vi "Tesla_Test.vi"() -> ()   [LabVIEW 2013]
uses:
  MM3_TESLA/Powerboard 1.0/Control/Command Enum.ctl
  <vilib>/Utility/NIReport.llb/NI_report.lvclass
  <vilib>/Utility/NIReport.llb/Append Report Text (str wrap).vi
  <vilib>/regexp/Match Regular Expression.xnode
panel:
  out "first subarray":string[](array[string])
  in  "Tab Control":T1(tab)
  in  "Protocol":bool
  in  "Text Base":bool
  in  "Network":bool
  in  "Commence":bool
  out "IP address":i32
  out "offset past match":i32
  out "concatenated string":string
  out "Ping Cout":i32
  in  "file path":path=path "C:/Users/barddya/Desktop/Tesla/List_of_IPs.txt"
  out "Hex 5":bool
  out "Hex 4":bool
  out "Hex 3":bool
  out "Hex 2":bool
  out "Hex 1":bool
  out "Percent 5":dbl
  out "Percent 4":dbl
  out "Percent 3":dbl
  out "Percent 2":dbl
  out "Percent 1":dbl
  out "Voltage 5":dbl
  out "Voltage 4":dbl
  out "Voltage 3":dbl
  out "Voltage 2":dbl
  out "Voltage 1":dbl
  out "Pass/Fail1 5":bool
  out "Pass/Fail1 4":bool
  out "Pass/Fail1 3":bool
  out "Pass/Fail1 2":bool
  out "Pass/Fail1":bool
  in  "Fast Stop":bool=TRUE
  in  "Don press continue":bool
  out "All Test Parameters":T2(array[cluster])
  # "Pass/Fail"
  # "Voltage"
  # "Precent"
  # "Is Hex"
  # "Results"
  # "Response 1"
  # "Response 2"
  # "Response 3"
  # "Response 4"
  # "Response 5"
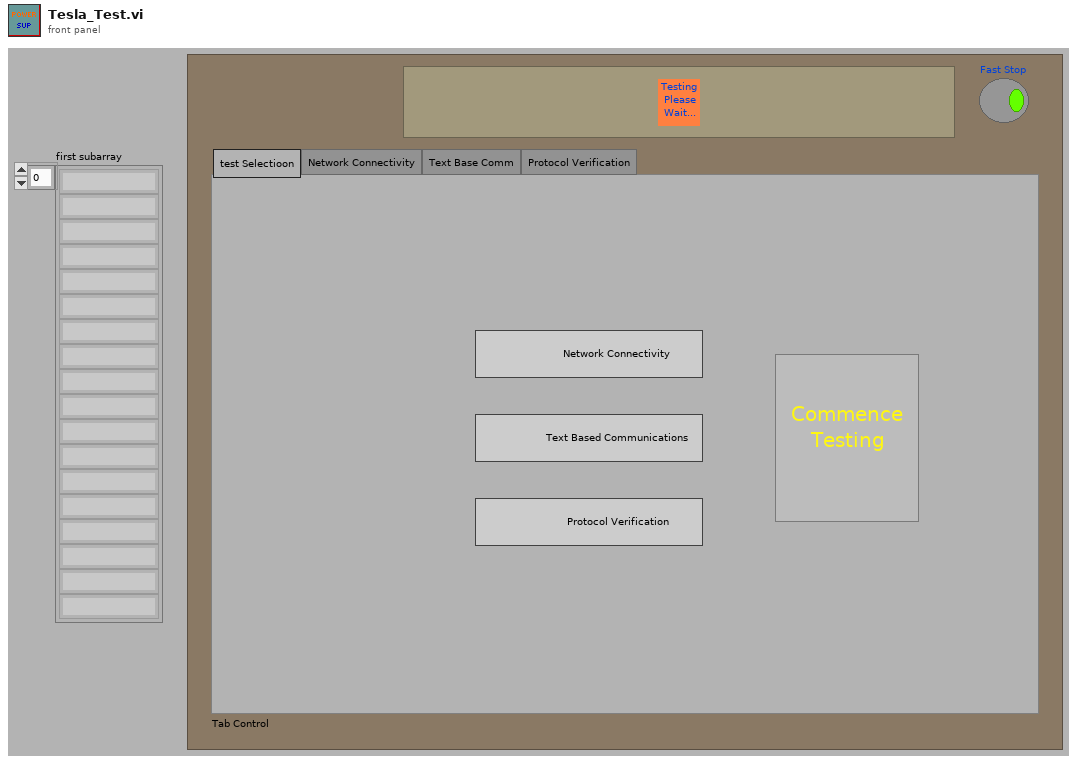
[diagram p1: front panel]
types:
  T1 = enum32{"test Selectioon", "Network Connectivity", "Text Base Comm", "Protocol Verification"}
  T2 = cluster{"[0]":string, "[1]":string, "[2]":string, "[3]":string, "[4]":string, "[5]":string, "[6]":string, "[7]":string, "[8]":string, "[9]":string, "[10]":string, "[11]":string, "[12]":string}[]
  T3 = typedef "Command Enum.ctl" = enum16{"Scan Serial", "set ports", "init devices", "nominal harvest", "basic functionality", "nominal supercap", "supercap balancing", "low harvest low load", "low harvest_supercap", "low supercap", "low suparcap low load", "low supercap high load", "supercap charge lowcap low p", "supercap charge high cap L.P", "PWM feedback", "supercap charge high P", "high harvest low load", "full power_overload", "full power high voltage", "display results", "Stop"}
  T4 = enum16{"open", "replace", "create", "open or create", "replace or create", "replace or create with confirmation"}
  T5 = cluster{"Charset (-1)":i16, "Weight (-1)":i16, "Name":string, "Size":string}
  T6 = enum16{"Standard Report", "HTML", "Word", "Excel"}
  T7 = cluster{"[0]":string, "[1]":string, "[2]":string, "[3]":string, "[4]":string, "[5]":string, "[6]":string, "[7]":string, "[8]":string, "[9]":string, "[10]":string, "[11]":string, "[12]":string}
  T8 = cluster{"output state":bool, "Device ID":i32, "Set CC current":dbl}
  T9 = enum16{"Left Button", "Center Button", "Right Button", "Window Close"}
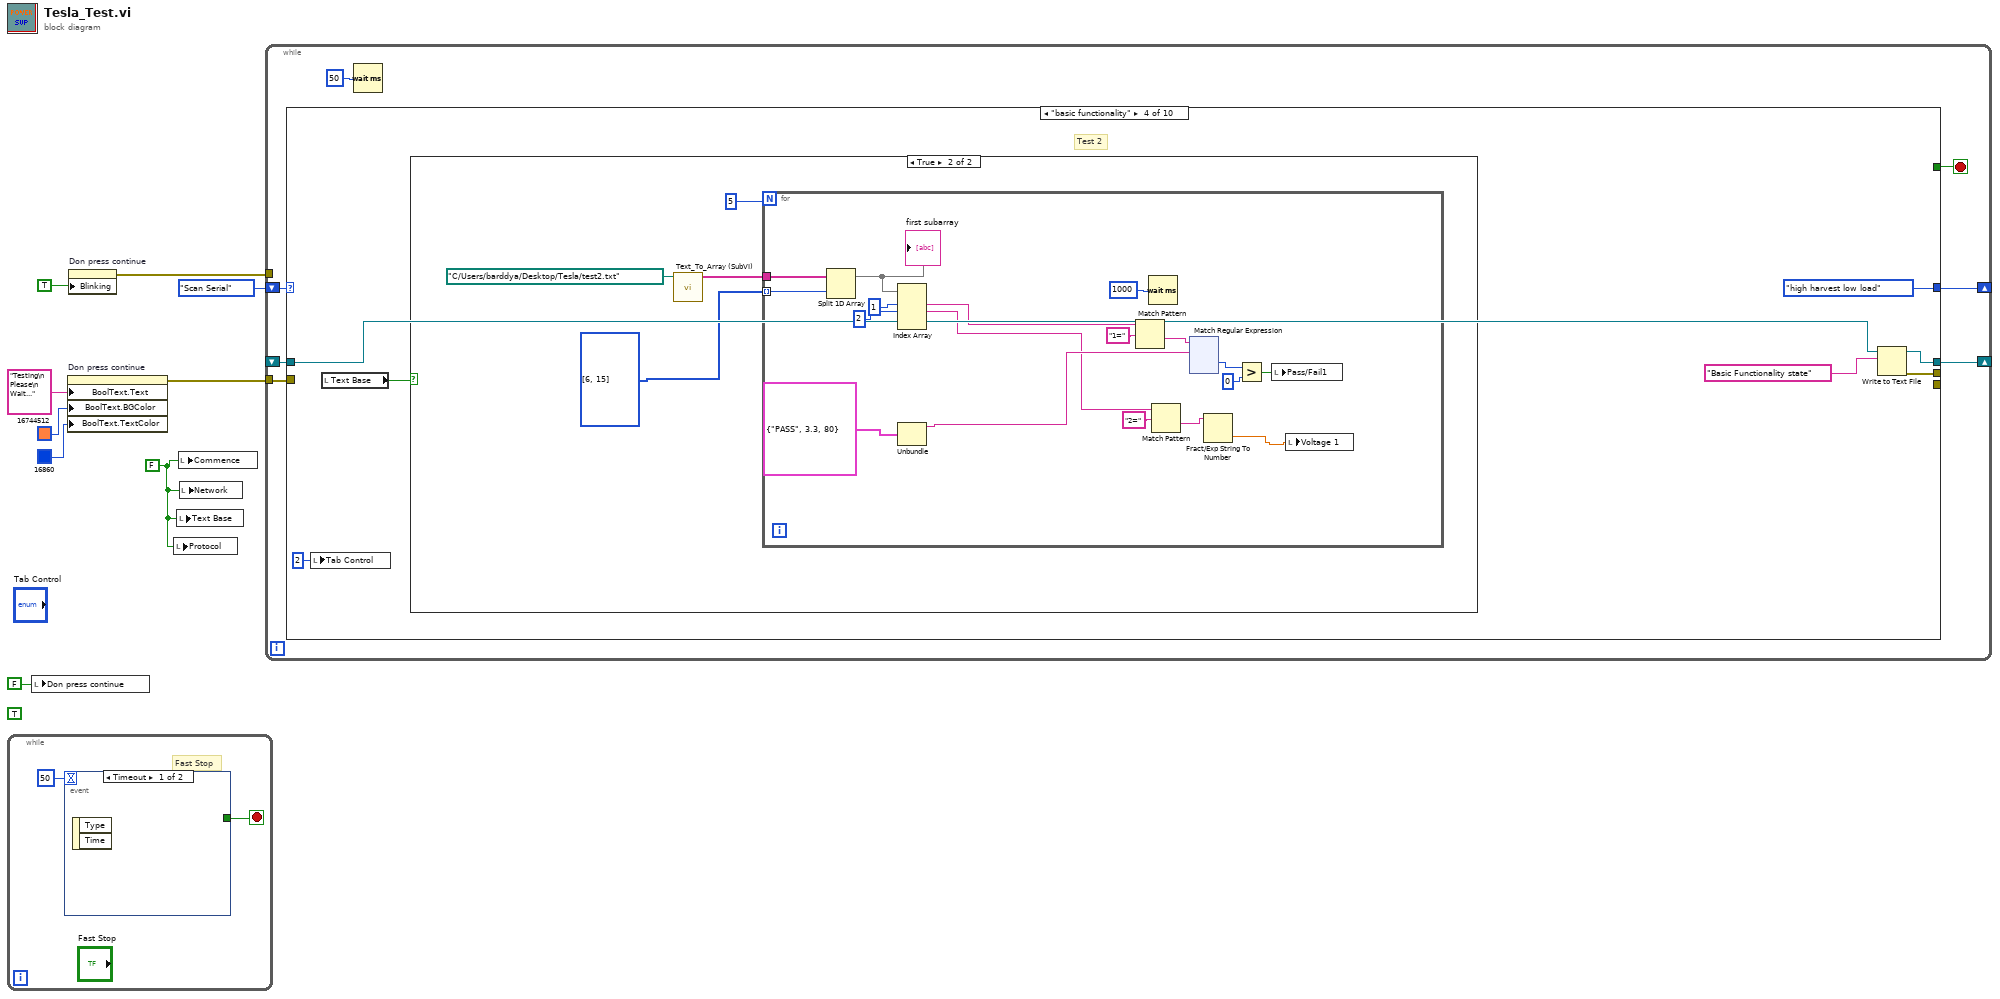
[diagram p0: block diagram]
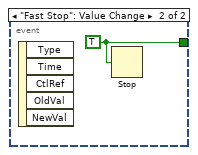
[diagram p2: hidden frame]
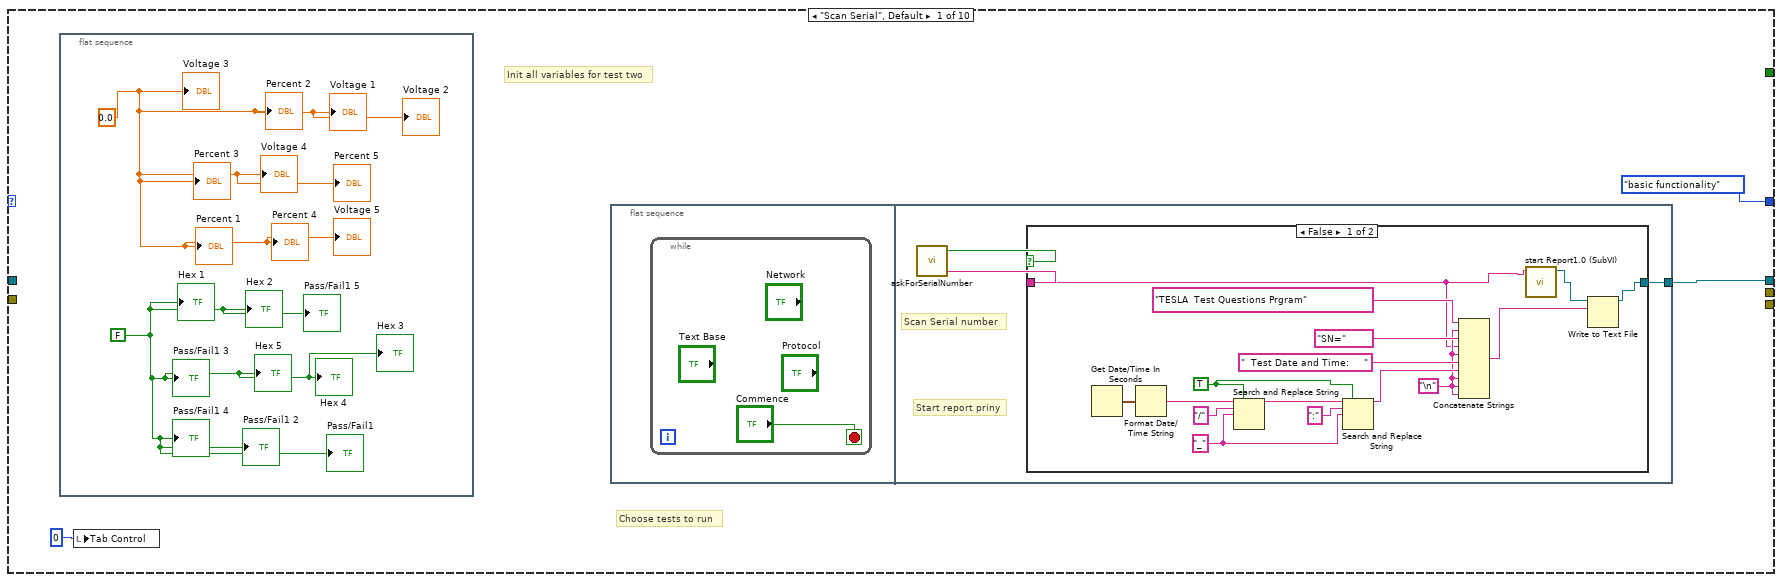
[diagram p3: hidden frame]
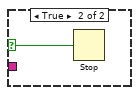
[diagram p4: hidden frame]
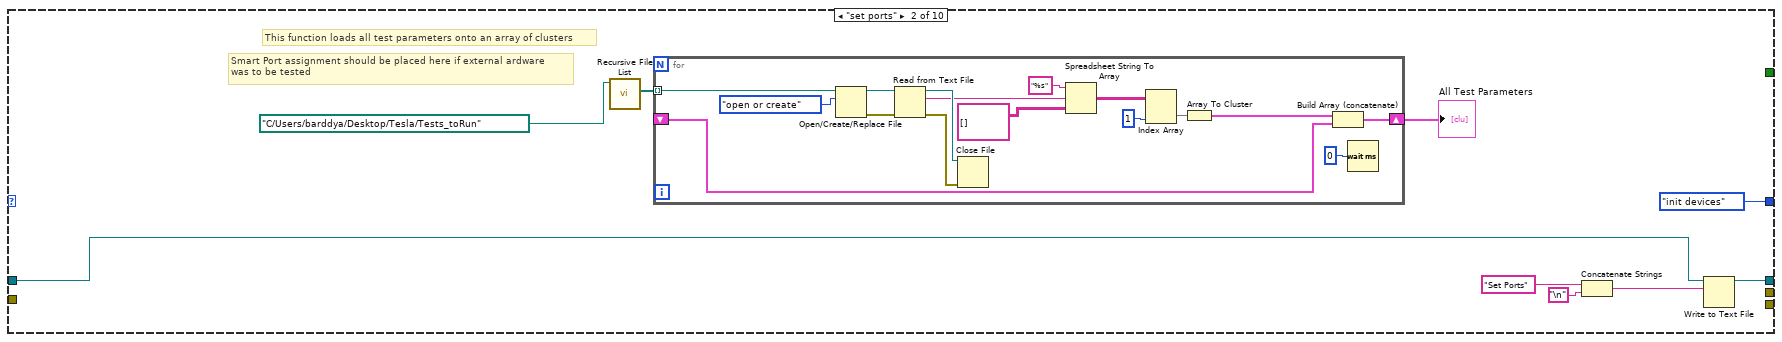
[diagram p5: hidden frame]
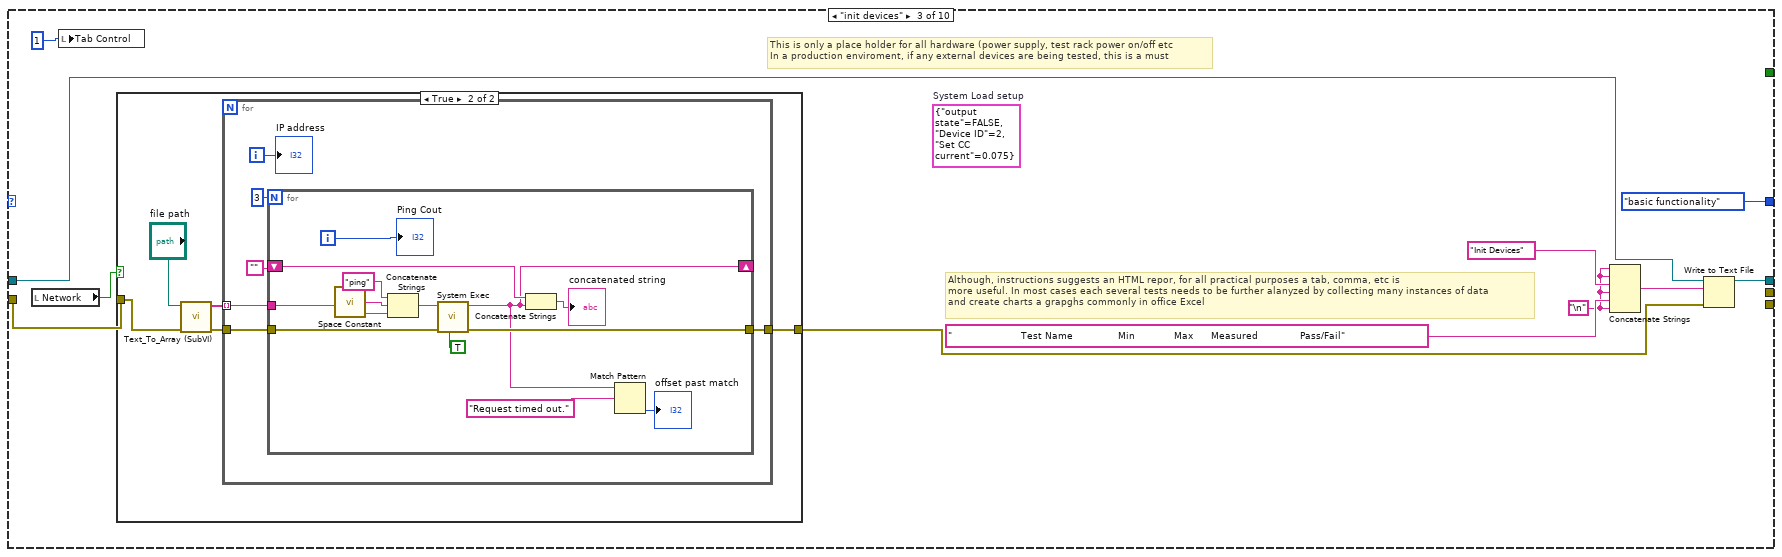
[diagram p6: hidden frame]
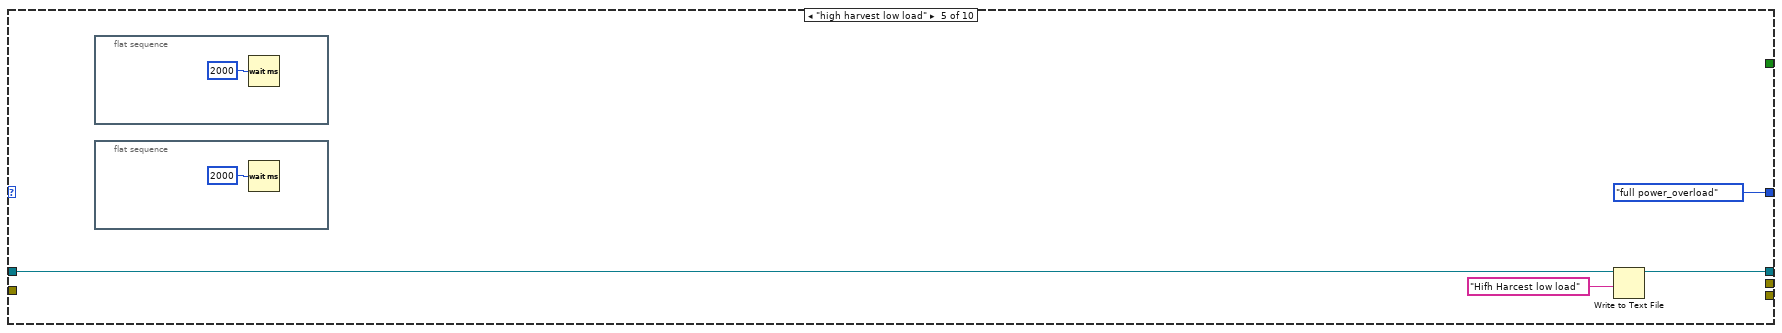
[diagram p9: hidden frame]
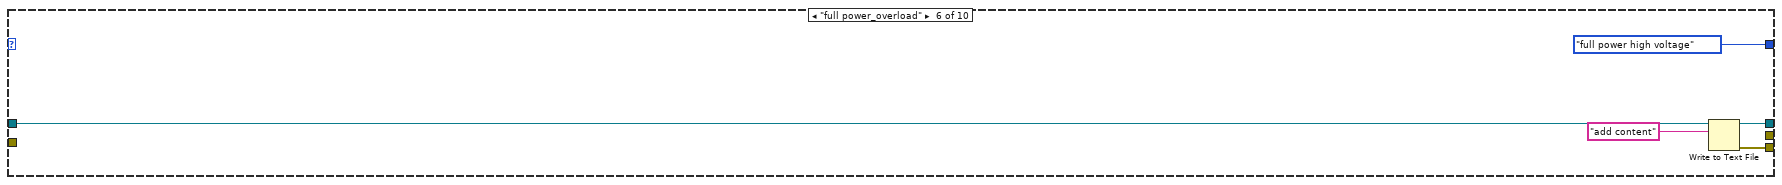
[diagram p10: hidden frame]
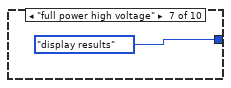
[diagram p11: hidden frame]
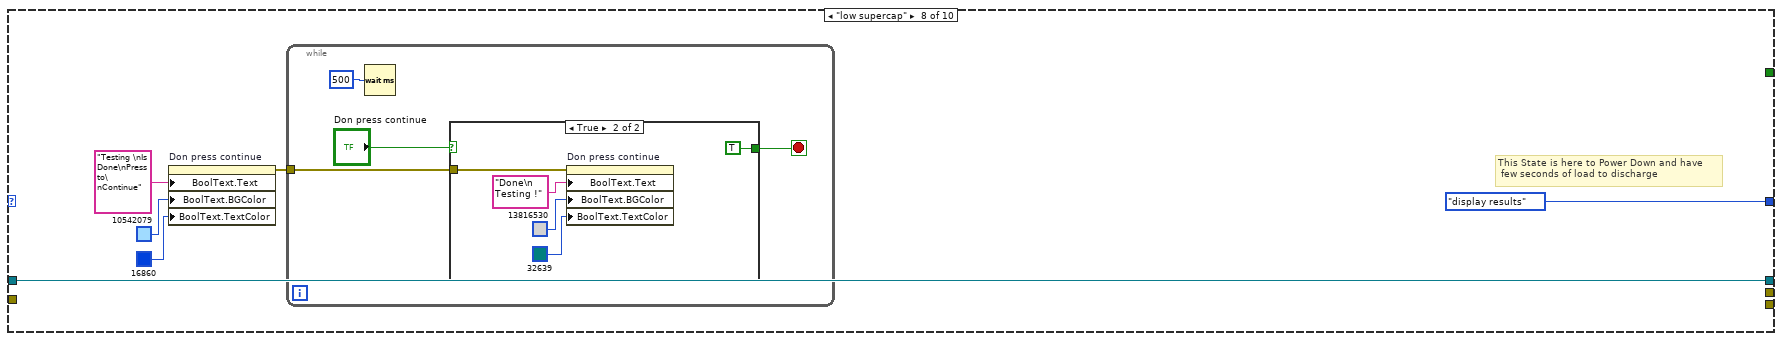
[diagram p12: hidden frame]
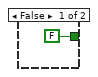
[diagram p13: hidden frame]
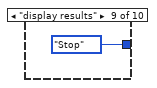
[diagram p14: hidden frame]
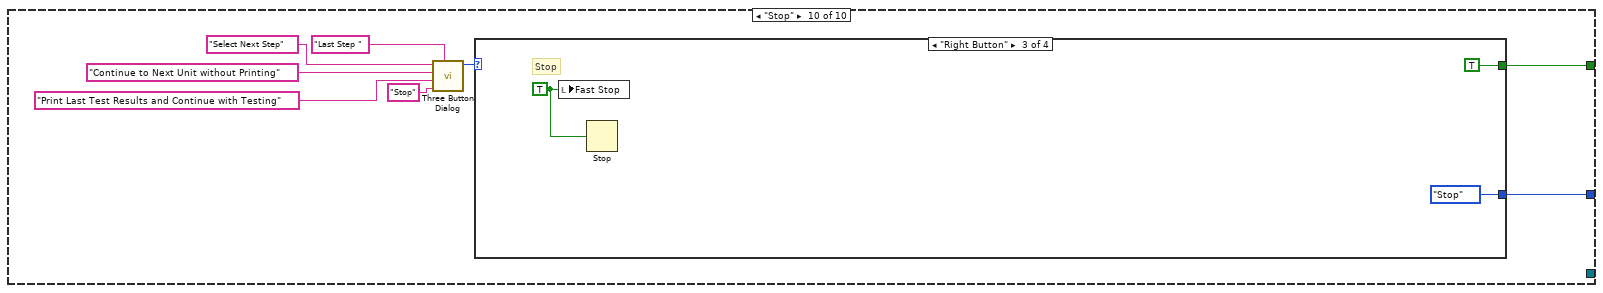
[diagram p15: hidden frame]
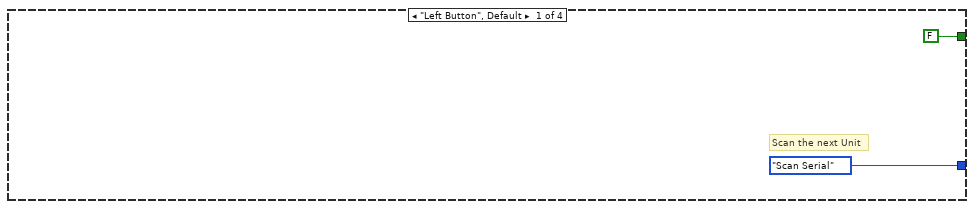
[diagram p16: hidden frame]
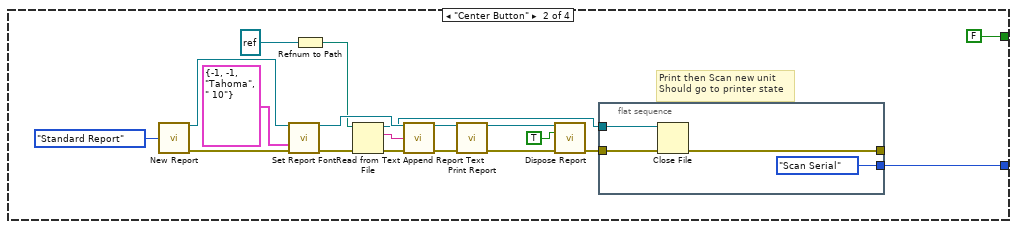
[diagram p17: hidden frame]
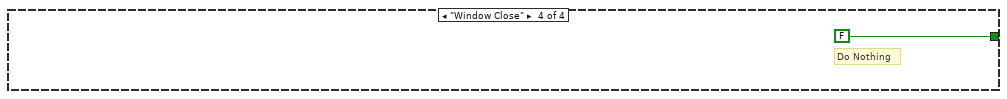
[diagram p18: hidden frame]
diagram:
  w1 = FALSE
  (unwired) TRUE
  n1 = while {
    stop <- w10 stop-if-true
    # "Fast Stop"
    n2 = event shown="[0] Timeout" {
      selector: _ -> [_ _]
      dyn-events: _ -> [_ _]
      timeout: 50 -> [_ _]
      tunnel: [_ w12] -> w10
      event Timeout {
        n3 = event-data() -> ()  [unwired: 1 in, 2 out]
      }
      event "Fast Stop": Value Change {
        w12 = TRUE
        n4 = event-data() -> ()  [unwired: 1 in, 5 out]
        n5 = Stop(stop? (T)=w12) -> ()
      }
    }
  }
  n6 = local write "Don press continue"(FALSE) -> ()
  n7 = property on="Don press continue" class="Bool (strict)"("BoolText.Text"="Testing\n Please\n Wait...", "BoolText.BGColor"=u32 16744512, "BoolText.TextColor"=u32 16860) -> (error out=w7:errorcluster)  [unwired: 2 in, 1 out]
  n8 = property on="Don press continue" class="Bool (strict)"("Blinking"=TRUE) -> (error out=w3:errorcluster)  [unwired: 2 in, 1 out]
  n9 = local write "Protocol"(w1) -> ()
  n10 = local write "Text Base"(w1) -> ()
  n11 = local write "Commence"(w1) -> ()
  n12 = local write "Network"(w1) -> ()
  n13 = while {
    shift-right: [w18] -> _
    shift-left: Command_Enum."Scan Serial" ("Command Enum") -> [w19]
    tunnel: w7 -> [w15]
    tunnel: w3 -> [_]
    shift-right: [w14] -> _
    shift-left: _ -> [w13]
    stop <- w17 stop-if-true
    n14 = case shown="\"basic functionality\"" w19 {
      tunnel: [Command_Enum."basic functionality" ("Command Enum") Command_Enum."init devices" ("Command Enum") Command_Enum."basic functionality" ("Command Enum") Command_Enum."high harvest low load" ("Command Enum") Command_Enum."full power_overload" ("Command Enum") Command_Enum."full power high voltage" ("Command Enum") Command_Enum."display results" ("Command Enum") Command_Enum."display results" ("Command Enum") Command_Enum."Stop" ("Command Enum") w280] -> w18
      tunnel: [_ _ _ _ _ _ _ _ _ w279] -> w17
      tunnel: w15 -> [_ _ w74 _ _ _ _ _ _ _]
      tunnel: [w21 w47 w79 w111 w252 w258 _ w262 _ _] -> w14
      tunnel: w13 -> [_ w46 w78 w110 w250 w256 _ w262 _ _]
      tunnel: [_ _ _ w112 _ _ _ _ _ _] -> _
      tunnel: [_ _ _ _ _ w259 _ _ _ _] -> _
      frame "Scan Serial", Default {
        # "Choose tests to run"
        # "Init all variables for test two"
        n15 = flat-sequence {
          frame #0 {
            w23 = FALSE
            w24 = 0.0
            "Voltage 5" <- w24
            "Percent 5" <- w24
            "Voltage 3" <- w24
            "Voltage 4" <- w24
            "Voltage 2" <- w24
            "Percent 4" <- w24
            "Percent 3" <- w24
            "Voltage 1" <- w24
            "Percent 2" <- w24
            "Percent 1" <- w24
            "Pass/Fail1 5" <- w23
            "Hex 5" <- w23
            "Pass/Fail1 3" <- w23
            "Pass/Fail1 4" <- w23
            "Pass/Fail1" <- w23
            "Hex 3" <- w23
            "Hex 4" <- w23
            "Hex 2" <- w23
            "Hex 1" <- w23
            "Pass/Fail1 2" <- w23
          }
        }
        n16 = local write "Tab Control"(0) -> ()
        n17 = flat-sequence {
          tunnel: [w26] -> w21
          frame #0 {
            n18 = while {
              stop <- "Commence" stop-if-true
            }
          }
          frame #1 {
            # "Start report priny"
            # "Scan Serial number"
            n19 = call "askForSerialNumber.vi"() -> ("Stop"=w28:bool, "Serial Number scanned"=w27:string)  [unwired: 1 in, 1 out]
            n20 = case shown="False" w28 {
              selector: w28 -> [_ w45]
              tunnel: w27 -> [w32 _]
              tunnel: [w30 _] -> w26
              frame False {
                w33 = "\n"
                w42 = TRUE ("replace all? (F)")
                w41 = "_"
                n21 = Get Date/Time In Seconds() -> (seconds since 1Jan1904=w36:timestamp)
                n22 = Format Date/Time String(seconds (now)=w36) -> (date/time string=w37:string)  [unwired: 2 in]
                n23 = Search and Replace String(replace all?=w42, input string=w37, search string="/", replace string=w41) -> (result string=w39:string)  [unwired: 4 in, 3 out]
                n24 = Search and Replace String(replace all?=w42, input string=w39, search string=":", replace string=w41) -> (result string=w44:string)  [unwired: 4 in, 3 out]
                n25 = Concatenate Strings("TESLA  Test Questions Prgram", w33, "SN=", w32, w33, "  Test Date and Time:     ", w44, w33, w33, w33) -> (w29:string)
                n26 = call "start Report1.0 (SubVI).vi"("Serial Number"=w32) -> ("Byte Stream File out"=w31:refnum<file>)  [unwired: 9 in, 1 out]
                n27 = Write to Text File(file (use dialog)=w31, text=w29) -> (refnum out=w30:refnum<file>)  [unwired: 2 in, 2 out]
              }
              frame True {
                n28 = Stop(stop? (T)=w45) -> ()
              }
            }
          }
        }
      }
      frame "set ports" {
        # "Smart Port assignment should be placed here if external ardware \nwas to be tested"
        # "This function loads all test parameters onto an array of clusters"
        n29 = call <vilib>:"Recursive File List.vi"("Folder Path"=path "C:/Users/barddya/Desktop/Tesla/Tests_toRun") -> ("All Files in Dir"=w53:path[])  [unwired: 6 in, 4 out]
        n30 = for {
          tunnel: w53 -> [w62] mode=indexing
          shift-right: [w59] -> w51
          shift-left: _ -> [w58]
          n31 = Open/Create/Replace File(file path (use dialog)=w62, operation (0:open)=T4."open or create") -> (refnum out=w66:refnum<file>, error out=w67:errorcluster)  [unwired: 4 in, 1 out]
          n32 = Read from Text File(file (use dialog)=w66, error in=w67) -> (refnum out=w70:refnum<file>, text=w65:string, error out=w69:errorcluster)  [unwired: 2 in, 1 out]
          n33 = Close File(refnum=w70, error in=w69) -> ()  [unwired: 2 out]
          n34 = Spreadsheet String To Array(format string="%s", spreadsheet string=w65, array type (2D Dbl)=string[][] []) -> (array=w56:string[][])  [unwired: 1 in]
          n35 = Index Array(array=w56, index (col)=1) -> (element=w55:string[])  [unwired: 1 in]
          n36 = Array To Cluster(array=w55) -> (cluster=w60:T7)
          n37 = Build Array (concatenate)(w60, w58) -> (w59:T2)
          n38 = Wait (ms)(milliseconds to wait=0) -> ()  [unwired: 1 out]
        }
        "All Test Parameters" <- w51
        n39 = Concatenate Strings("Set Ports", "\n") -> (w49:string)
        n40 = Write to Text File(file (use dialog)=w46, text=w49) -> (refnum out=w47:refnum<file>)  [unwired: 2 in, 2 out]
      }
      frame "init devices" {
        w75 = "\n"
        (unwired) T8 {"output state"=FALSE, "Device ID"=2, "Set CC current"=0.075}  # System Load setup
        # "Although, instructions suggests an HTML repor, for all practical purposes a tab, comma, etc is \nmore useful. In most cases each several tests needs to be further alanyzed by collecting many instances of data \nand create charts a grapghs commonly in office Excel"
        # "This is only a place holder for all hardware (power supply, test rack power on/off etc\nIn a production enviroment, if any external devices are being tested, this is a must"
        n41 = local read "Network"() -> (w71:bool)
        n42 = local write "Tab Control"(1) -> ()
        n43 = case shown="True" w71 {
          tunnel: w74 -> [w82 w84]
          tunnel: [w82 w83] -> w73
          frame False {
          }
          frame True {
            n44 = call "Text_To_Array (SubVI).vi"("error in (no error)"=w84, "file path"="file path") -> ("error out"=w86:errorcluster, "Array"=w87:string[])  [unwired: 7 in, 1 out]
            n45 = for {
              tunnel: w87 -> [w91] mode=indexing
              tunnel: w86 -> [w93]
              tunnel: [w92] -> w83
              i -> [w89]
              n46 = for {
                N: 3 -> [_]
                tunnel: w93 -> [w106]
                tunnel: [w105] -> w92
                tunnel: w91 -> [w103]
                shift-right: [w96] -> _
                shift-left: "" -> [w98]
                i -> [w99]
                n47 = call <vilib>:"Space Constant.vi"() -> ("String"=w101:string)
                n48 = Concatenate Strings("ping", w101, w103) -> (w104:string)
                n49 = call <vilib>:"System Exec.vi"("run minimized? (F)"=TRUE, "error in (no error)"=w106, "command line"=w104) -> ("error out"=w105:errorcluster, "standard output"=w96:string)  [unwired: 5 in, 2 out]
                n50 = Concatenate Strings(w98, w96) -> (→"concatenated string":string)
                n51 = Match Pattern(string=w96, regular expression="Request timed out." ("search string/char (-)")) -> (offset past match=→"offset past match":i32)  [unwired: 1 in, 3 out]
                "Ping Cout" <- w99
              }
              "IP address" <- w89
            }
          }
        }
        n52 = Concatenate Strings(w75, w75, "Init Devices", w75, "                       Test Name               Min             Max      Measured              Pass/Fail", w75) -> (w80:string)
        n53 = Write to Text File(file (use dialog)=w78, text=w80, error in=w73) -> (refnum out=w79:refnum<file>)  [unwired: 1 in, 2 out]
      }
      frame "basic functionality" {
        # "Test 2"
        n54 = local write "Tab Control"(2) -> ()
        n55 = local read "Text Base"() -> (w108:bool)
        n56 = case shown="True" w108 {
          frame False {
          }
          frame True {
            n57 = call "Text_To_Array (SubVI).vi"("file path"=path "C:/Users/barddya/Desktop/Tesla/test2.txt") -> ("Array"=w116:string[])  [unwired: 8 in, 2 out]
            n58 = for {
              N: 5 -> [_]
              tunnel: w116 -> [w135]
              tunnel: i32[] [6, 15] -> [w129] mode=indexing
              n59 = Split 1D Array(array=w135, index=w129) -> (first subarray=w128:string[])  [unwired: 1 out]
              "first subarray" <- w128
              n60 = Index Array(array=w128, index #1=1, index #2=2) -> (element #1=w122:string, element #2=w118:string)  [unwired: 2 in, 2 out]
              n61 = Unbundle(cluster{string, dbl, i32} {"PASS", 3.3, 80}) -> (w133:string)  [unwired: 2 out]
              n62 = Match Pattern(string=w122, regular expression="1=") -> (after substring=w130:string)  [unwired: 1 in, 3 out]
              n63 = Wait (ms)(milliseconds to wait=1000) -> ()  [unwired: 1 out]
              n64 = Match Pattern(string=w118, regular expression="2=") -> (after substring=w121:string)  [unwired: 1 in, 3 out]
              n65 = xnode "Match Regular Expression"("input string"=w130, "regular expression"=w133) -> ("offset past match"=w126:i32)  [unwired: 4 in, 4 out]
              n66 = Fract/Exp String To Number(string=w121) -> (number=w120:dbl)  [unwired: 3 in, 1 out]
              n67 = Greater?(x=w126, y=0) -> (0:w124:bool)
              n68 = local write "Pass/Fail1"(w124) -> ()
              n69 = local write "Voltage 1"(w120) -> ()
            }
          }
        }
        n70 = Write to Text File(file (use dialog)=w110, text="Basic Functionality state") -> (refnum out=w111:refnum<file>, error out=w112:errorcluster)  [unwired: 2 in, 1 out]
      }
      frame "high harvest low load" {
        n71 = flat-sequence {
          frame #0 {
            n72 = Wait (ms)(milliseconds to wait=2000) -> ()  [unwired: 1 out]
          }
        }
        n73 = flat-sequence {
          frame #0 {
            n74 = Wait (ms)(milliseconds to wait=2000) -> ()  [unwired: 1 out]
          }
        }
        n75 = Write to Text File(file (use dialog)=w250, text="Hifh Harcest low load") -> (refnum out=w252:refnum<file>)  [unwired: 2 in, 2 out]
      }
      frame "full power_overload" {
        n76 = Write to Text File(file (use dialog)=w256, text="add content") -> (refnum out=w258:refnum<file>, error out=w259:errorcluster)  [unwired: 2 in, 1 out]
      }
      frame "full power high voltage" {
      }
      frame "low supercap" {
        # "This State is here to Power Down and have\n few seconds of load to discharge"
        n77 = property on="Don press continue" class="Bool (strict)"("BoolText.Text"="Testing \nIs Done\nPress to\nContinue", "BoolText.BGColor"=u32 10542079, "BoolText.TextColor"=u32 16860) -> (error out=w266:errorcluster)  [unwired: 2 in, 1 out]
        n78 = while {
          tunnel: w266 -> [w269]
          stop <- w268 stop-if-true
          n79 = Wait (ms)(milliseconds to wait=500) -> ()  [unwired: 1 out]
          n80 = case shown="True" "Don press continue" {
            tunnel: [FALSE TRUE] -> w268
            tunnel: w269 -> [_ w274]
            frame False {
            }
            frame True {
              n81 = property on="Don press continue" class="Bool (strict)"(error in=w274, "BoolText.Text"="Done\n Testing !", "BoolText.BGColor"=u32 13816530, "BoolText.TextColor"=u32 32639) -> ()  [unwired: 1 in, 2 out]
            }
          }
        }
      }
      frame "display results" {
      }
      frame "Stop" {
        n82 = call <vilib>:"Three Button Dialog.vi"("Window Title (\"\")"="Last Step " ("Window Title (\"\")"), "Right Button Text (\"Cancel\")"="Stop" ("Window Title (\"\")"), "Center Button Text (\"No\")"="Print Last Test Results and Continue with Testing" ("Window Title (\"\")"), "Left Button Text (\"Yes\")"="Continue to Next Unit without Printing" ("Window Title (\"\")"), "message"="Select Next Step" ("Window Title (\"\")")) -> ("Which Button?"=w286:T9)  [unwired: 6 in]
        n83 = case shown="\"Right Button\"" w286 {
          tunnel: [Command_Enum."Scan Serial" ("Command Enum") w291 Command_Enum."Stop" ("Command Enum") _] -> w280
          tunnel: [FALSE FALSE TRUE FALSE] -> w279
          frame "Left Button", Default {
            # "Scan the next Unit"
          }
          frame "Center Button" {
            # "Print then Scan new unit\nShould go to printer state"
            n84 = call <vilib>:"New Report.vi"("report type"=T6."Standard Report") -> ("report out"=w304:refnum<class "NI_report.lvclass">, "error out"=w305:errorcluster)  [unwired: 13 in]
            n85 = call-dynamic "Set Report Font.vi"("report in"=w304, "font settings"=T5 {"Charset (-1)"=-1, "Weight (-1)"=-1, "Name"="Tahoma", "Size"=" 10"}, "error in (no error)"=w305) -> ("report out"=w303:refnum<class "NI_report.lvclass">, "error out"=w302:errorcluster)  [unwired: 10 in, 1 out]
            n86 = Refnum to Path(1:refnum<file> refnum ("refnum")) -> (0:w290:path)
            n87 = Read from Text File(file (use dialog)=w290, error in=w302) -> (refnum out=w292:refnum<file>, text=w301:string, error out=w300:errorcluster)  [unwired: 2 in, 1 out]
            n88 = call-poly <vilib>:"Append Report Text.vi"("report in"=w303, "text"=w301, "error in (no error)"=w300) -> ("report out"=w299:refnum<class "NI_report.lvclass">, "error out"=w296:errorcluster)  [unwired: 9 in, 2 out]
            n89 = call-dynamic "Print Report.vi"("report in"=w299, "error in (no error)"=w296) -> ("report out"=w297:refnum<class "NI_report.lvclass">, "error out"=w298:errorcluster)  [unwired: 12 in]
            n90 = call-dynamic "Dispose Report.vi"("report in"=w297, "wait until printing completed? (T)"=TRUE, "error in (no error)"=w298) -> ("error out"=w293:errorcluster)  [unwired: 12 in]
            n91 = flat-sequence {
              tunnel: w293 -> [w311]
              tunnel: [w310] -> _
              tunnel: w292 -> [w309]
              tunnel: [Command_Enum."Scan Serial" ("Command Enum")] -> w291
              frame #0 {
                n92 = Close File(refnum=w309, error in=w311) -> (error out=w310:errorcluster)  [unwired: 1 out]
              }
            }
          }
          frame "Right Button" {
            w312 = TRUE
            # "Stop"
            n93 = local write "Fast Stop"(w312) -> ()
            n94 = Stop(stop? (T)=w312) -> ()
          }
          frame "Window Close" {
            # "Do Nothing"
          }
        }
      }
    }
    n95 = Wait (ms)(milliseconds to wait=50) -> ()  [unwired: 1 out]
  }
